vi "Read Current Setpoint.vi"(8 "error in":errorcluster, 11 "Current Control in":refnum<class "Current Control.lvclass">) -> (0 "error out":errorcluster, 1 "Changed or First Call?":bool, 2 "Current Setpoint":dbl, 3 "Current Control out":refnum<class "Current Control.lvclass">)   [LabVIEW 2023, in "Current Control.lvclass"]
uses:
  Current Control.lvclass
  Current Control.lvclass/Current Control.ctl
  <vilib>/ADAS Replay HIL/Channels/Tag Wrapper/Tag Wrapper.lvlib
  49ccd0c4-676c-49c2-8dbb-76c3f60c238e.vi
  <vilib>/ADAS Replay HIL/Channels/Tag Wrapper/Polymorphic/Read Channel (Double).vi
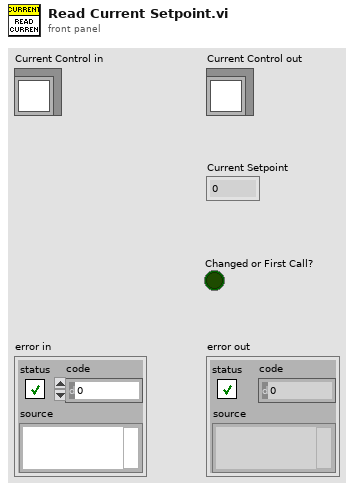
[diagram p1: front panel]
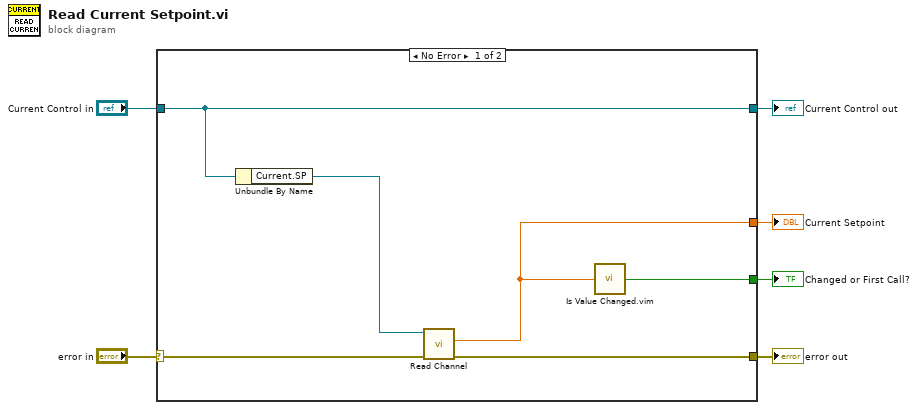
[diagram p0: block diagram]
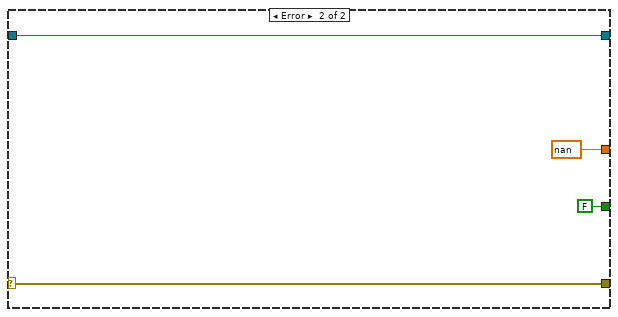
[diagram p2: hidden frame]
diagram:
  n1 = case shown="No Error" "error in" {
    selector: "error in" -> [w10 w16]
    tunnel: [w9 w16] -> w5
    tunnel: [w12 w15] -> w3
    tunnel: "Current Control in" -> [w12 w15]
    tunnel: [w8 nan] -> w1
    tunnel: [w7 FALSE ("changed or first call?")] -> w2
    frame No Error {
      n2 = Unbundle By Name(w12) -> ("Current.SP"=w11:refnum<k21>)
      n3 = call-poly <vilib>:"Read Channel.vi"("error in"=w10, "ADAS HIL Channel in"=w11) -> ("error out"=w9:errorcluster, "Value out"=w8:dbl)  [unwired: 6 in, 2 out]
      n4 = call "Is Value Changed.vim"("value"=w8) -> ("changed or first call?"=w7:bool)
    }
    frame Error {
    }
  }
  "error out" <- w5
  "Current Control out" <- w3
  "Changed or First Call?" <- w2
  "Current Setpoint" <- w1
